vi "Test Boards_TASK.vi"() -> ()   [LabVIEW 2023]
doc: "See <b>Read_Me.html</b> in the <b>Board Testing</b> project for a detailed description of this VI."
uses:
  Common/Board Image.ctl
panel:
  out "Test Results":T2(array[cluster])
  # "Overview: Demonstrates a task-based solution to a board testing problem.\n\nSee Read_Me.html in the project for a detailed description of this VI."
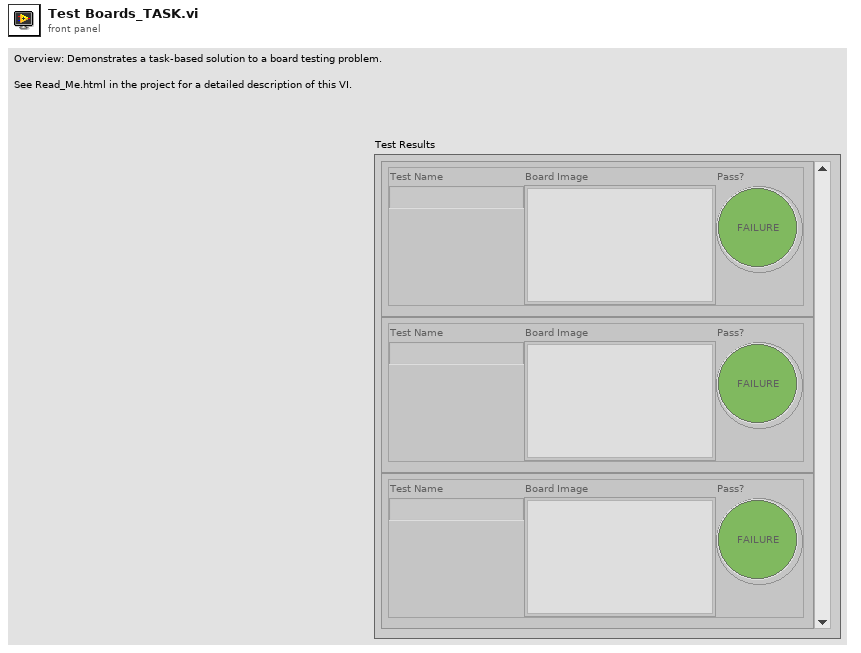
[diagram p1: front panel]
types:
  T1 = typedef "Board Image.ctl" = picture
  T2 = cluster{"Test Name":string, "Board Image":T1, "Pass?":bool}[]
  T3 = typedef "Assembly Line Input.ctl" = cluster{"board image":T1, "which board":T4}
  T4 = typedef "Board Type Enum.ctl" = enum16{"Basic DAQ Board", "Elite DAQ Board", "GPIB Board"}
  T5 = typedef "Pass Fail Boolean.ctl" = bool
  T6 = cluster{"test name":string, "board image":T1, "Pass?":T5}
  T7 = cluster{"test name":string, "board image":T1, "pass?":T5}
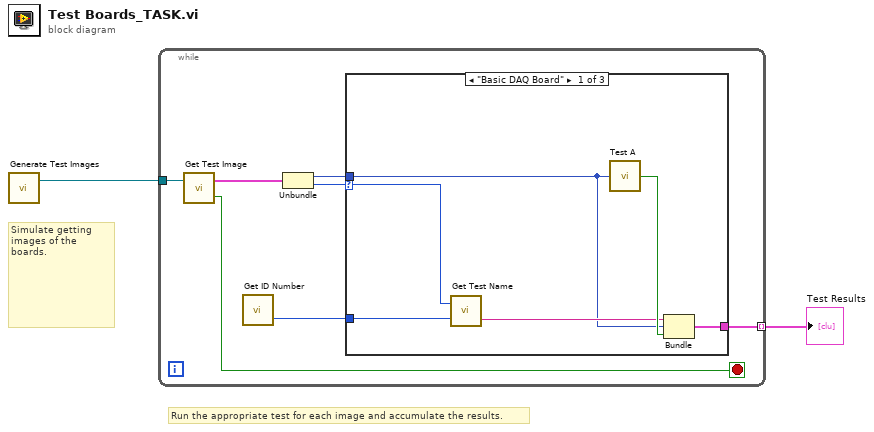
[diagram p0: block diagram]
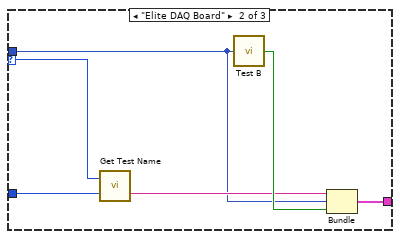
[diagram p2: hidden frame]
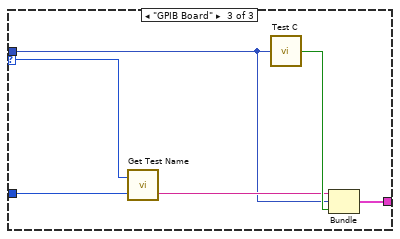
[diagram p3: hidden frame]
diagram:
  # "Run the appropriate test for each image and accumulate the results."
  # "Simulate getting images of the boards."
  n1 = call "Generate Test Images.vi"() -> ("queue out"=w2:refnum<queue>)  [unwired: 2 in, 1 out]
  n2 = while {
    tunnel: w2 -> [w9]
    tunnel: [w5] -> w1 mode=indexing
    stop <- w8 stop-if-true
    n3 = call "Get Test Image.vi"("queue in"=w9) -> ("no more images after this?"=w8:bool, "Assembly Line Image"=w7:T3)  [unwired: 1 in]
    n4 = call "Get ID Number.vi"() -> ("id number"=w3:u32)  [unwired: 2 in]
    n5 = Unbundle(w7) -> ("board image"=w4:T1, "which board"=w6:T4)
    n6 = case shown="\"Basic DAQ Board\"" w6 {
      selector: w6 -> [w15 w21 w27]
      tunnel: [w14 w20 w26] -> w5
      tunnel: w4 -> [w11 w17 w23]
      tunnel: w3 -> [w10 w16 w22]
      frame "Basic DAQ Board" {
        n7 = call "Get Test Name.vi"("id number"=w10, "which board"=w15) -> ("test name"=w12:string)  [unwired: 1 in]
        n8 = call "Test A.vi"("board image"=w11) -> ("Pass?"=w13:T5)
        n9 = Bundle("test name"=w12, "board image"=w11, "Pass?"=w13) -> (w14:T6)  [unwired: 1 in]
      }
      frame "Elite DAQ Board" {
        n10 = call "Get Test Name.vi"("id number"=w16, "which board"=w21) -> ("test name"=w18:string)  [unwired: 1 in]
        n11 = call "Test B.vi"("board image"=w17) -> ("pass?"=w19:T5)
        n12 = Bundle("test name"=w18, "board image"=w17, "pass?"=w19) -> (w20:T7)  [unwired: 1 in]
      }
      frame "GPIB Board" {
        n13 = call "Get Test Name.vi"("id number"=w22, "which board"=w27) -> ("test name"=w24:string)  [unwired: 1 in]
        n14 = call "Test C.vi"("board image"=w23) -> ("pass?"=w25:T5)
        n15 = Bundle("test name"=w24, "board image"=w23, "pass?"=w25) -> (w26:T7)  [unwired: 1 in]
      }
    }
  }
  "Test Results" <- w1
